vi "Default Settings.vi"(8 "error in (no error)":errorcluster, 11 "6 inch CAD Dispense in":refnum<class "6 inch CAD Dispense.lvclass">) -> (0 "error out":errorcluster, 3 "6 inch CAD Dispense out":refnum<class "6 inch CAD Dispense.lvclass">)   [LabVIEW 2019, in "6 inch CAD Dispense.lvclass"]
uses:
  6 inch CAD Dispense.lvclass
  C:/Users/HEP/Documents/Aerotech gantry/UCSB-Gantry-master-main/V5/Classes/Routine/Dispense/CAD Dispense/CAD Dispense.lvclass
  C:/Users/HEP/Documents/Aerotech gantry/UCSB-Gantry-master-main/V5/Classes/Routine/Dispense/Dispense.lvclass
  CAD Dispense.lvclass/CAD Dispense.ctl
  Read Glue Speed.vi
  Read Move Speed.vi
  CAD Dispense.lvclass
  Dispense.lvclass
panel:
  # "This Routine does not Accept Settings"
  # "This Routine Does not Accept Settings"
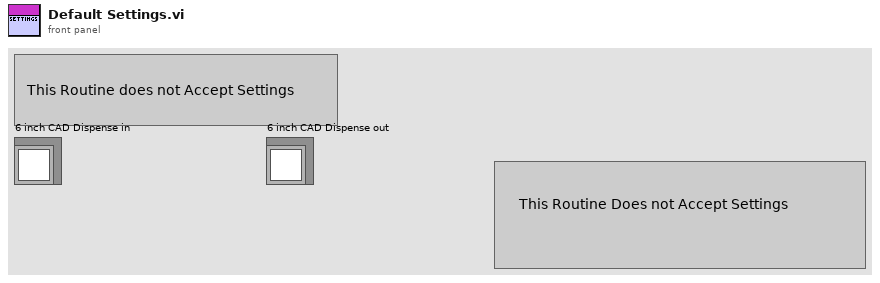
[diagram p1: front panel]
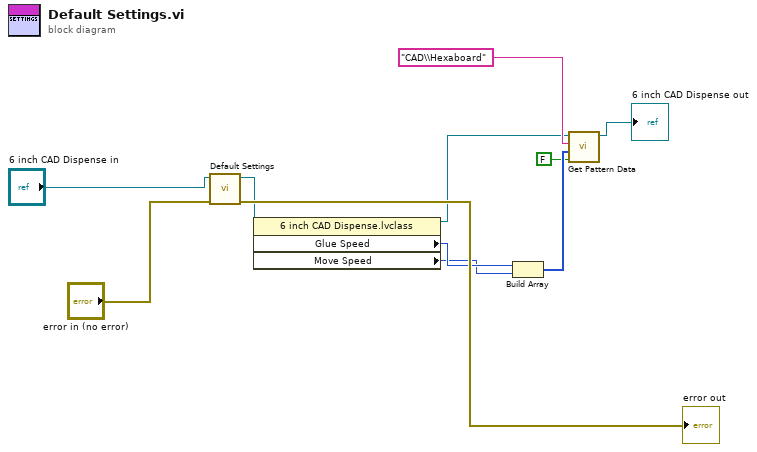
[diagram p0: block diagram]
diagram:
  n1 = call-parent "Default Settings.vi"("error in (no error)"="error in (no error)", "CAD Dispense in"="6 inch CAD Dispense in") -> ("error out"=→"error out":errorcluster, "CAD Dispense out"=w8:refnum<class "6 inch CAD Dispense.lvclass">)  [unwired: 8 in]
  n2 = property class="6 inch CAD Dispense.lvclass"(reference=w8) -> (reference out=w2:refnum<class "6 inch CAD Dispense.lvclass">, "Glue Speed"=w7:i32, "Move Speed"=w6:i32)  [unwired: 1 in, 1 out]
  n3 = Build Array "Build Array"(w7, w6) -> (w5:i32[])
  n4 = call "Get Pattern Data.vi"("Iterative?"=FALSE, "File Name"=w5, "Folder Name"="CAD\\Hexaboard", "Dispense.lvclass"=w2) -> ("Dispense Out"=→"6 inch CAD Dispense out":refnum<class "6 inch CAD Dispense.lvclass">)  [unwired: 7 in]
